vi "SECoP_dataDestroy.vi"(8 "error in (no error)":errorcluster, 10 "SECoP_dataPtr":T1 {"ptr64" format="%.0x"; "ptr32" format="%.0x"}, 11 "DLL path (in)":T2) -> (0 "error out":errorcluster, 3 "DLL path (out)":T2)   [LabVIEW 2023, in "SECoP.lvlib"]
doc: "Call <b>\"SECoP_dataDestroy.vi\"</b> to make references to this data value invalid and release memory.\nAfter call, references to this value will not be useable anymore and access function will return with an error.\n\n<b>DLL path</b> input and output of cluster from \"SECoP-Initialize.vi\"\n<b>SECoP_dataPtr</b> data to destroy"
uses:
  SECoP.lvlib
  SECoP-libraries.ctl
  SECoP-data.ctl
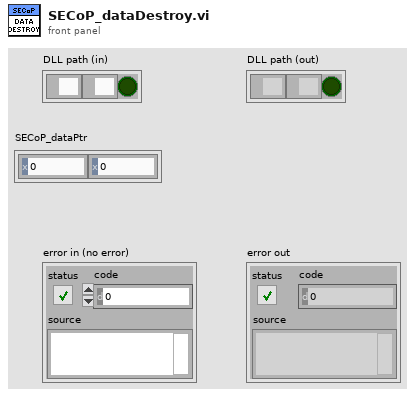
[diagram p1: front panel]
types:
  T1 = typedef "SECoP.lvlib/SECoP-data.ctl" = cluster{"ptr32":u32, "ptr64":u64}
  T2 = typedef "SECoP.lvlib/SECoP-libraries.ctl" = cluster{"serverDLL":path, "variantDLL":path, "cleanup_mode":bool}
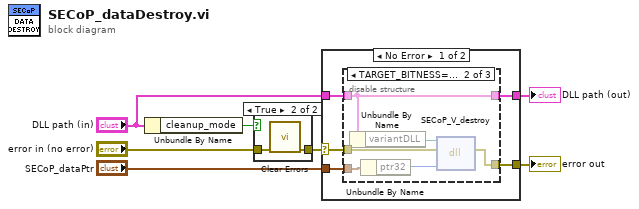
[diagram p0: block diagram]
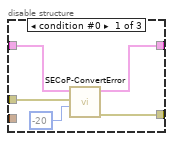
[diagram p3: hidden frame]
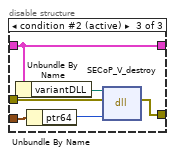
[diagram p4: hidden frame]
diagram:
  n1 = Unbundle By Name("DLL path (in)") -> ("cleanup_mode"=w5:bool)
  n2 = case shown="True" w5 {
    tunnel: "error in (no error)" -> [w8 w10]
    tunnel: [w8 w9] -> w3
    frame False {
    }
    frame True {
      n3 = call <vilib>:"Clear Errors.vi"("error in (no error)"=w10) -> ("error out"=w9:errorcluster)  [unwired: 5 in, 1 out]
    }
  }
  n4 = case shown="No Error" w3 {
    selector: w3 -> [w15 w33]
    tunnel: "DLL path (in)" -> [w14 w34]
    tunnel: [w12 w34] -> w7
    tunnel: [w13 w33] -> w6
    tunnel: "SECoP_dataPtr" -> [w11 _]
    frame No Error {
      n5 = disable-structure shown="TARGET_BITNESS==32" {
        disable-tunnel: w15 -> [w17 w26 w32]
        disable-tunnel: w14 -> [w20 w21 w27]
        disable-tunnel: [w18 w25 w31] -> w13
        disable-tunnel: [w19 w21 w27] -> w12
        disable-tunnel: w11 -> [_ w24 w30]
        frame condition #0 {
          n6 = call "SECoP-ConvertError.vi"("return code"=-20, "error in (no error)"=w17, "DLL path (in)"=w20) -> ("error out"=w18:errorcluster, "DLL path (out)"=w19:T2)  [unwired: 7 in]
        }
        frame condition #1 {
          n7 = Unbundle By Name(w21) -> ("variantDLL"=w22:path)
          n8 = Unbundle By Name(w24) -> ("ptr32"=w23:u32)
          n9 = dll-call lib="Z:/Praktische_Aufgaben/SECoP-LabVIEW2015/32bit/SECoP32.dll" fn="SECoP_V_destroy"(path in=w22, error in=w26, "data"=w23) -> (error out=w25:errorcluster)  [unwired: 3 in, 1 out]
        }
        frame condition #2 (active) {
          n10 = Unbundle By Name(w27) -> ("variantDLL"=w28:path)
          n11 = Unbundle By Name(w30) -> ("ptr64"=w29:u64)
          n12 = dll-call lib="Z:/Praktische_Aufgaben/SECoP-LabVIEW2015/32bit/SECoP32.dll" fn="SECoP_V_destroy"(path in=w28, error in=w32, "data"=w29) -> (error out=w31:errorcluster)  [unwired: 3 in, 1 out]
        }
      }
    }
    frame Error {
    }
  }
  "DLL path (out)" <- w7
  "error out" <- w6
